vi "New.vi"(8 "error in (no error)":errorcluster, 11 "reference in":refnum<class "TestSuite_InterfaceDelegation.lvclass">) -> (0 "error out":errorcluster, 3 "reference out":refnum<class "TestSuite_InterfaceDelegation.lvclass">)   [LabVIEW 2013, in "TestSuite_InterfaceDelegation.lvclass"]
uses:
  TestSuite_InterfaceDelegation.lvclass
  Test Cases/StringList_Delegations/StringList_Delegations.lvclass
  Test Cases/ObjectList_Delegations/ObjectList_Delegations.lvclass
  <vilib>/addons/_JKI Toolkits/VI Tester/TestCase.llb/TestCase.lvclass
  TestSuite_InterfaceDelegation.lvclass/TestSuite_InterfaceDelegation.ctl
  <vilib>/addons/_JKI Toolkits/VI Tester/TestSuite.llb/TestSuite.lvclass
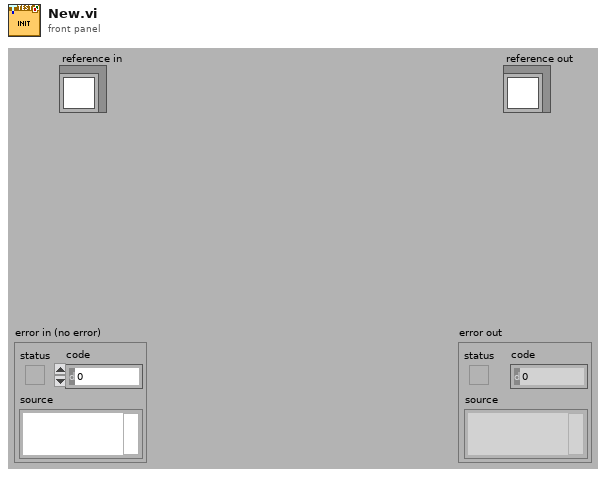
[diagram p1: front panel]
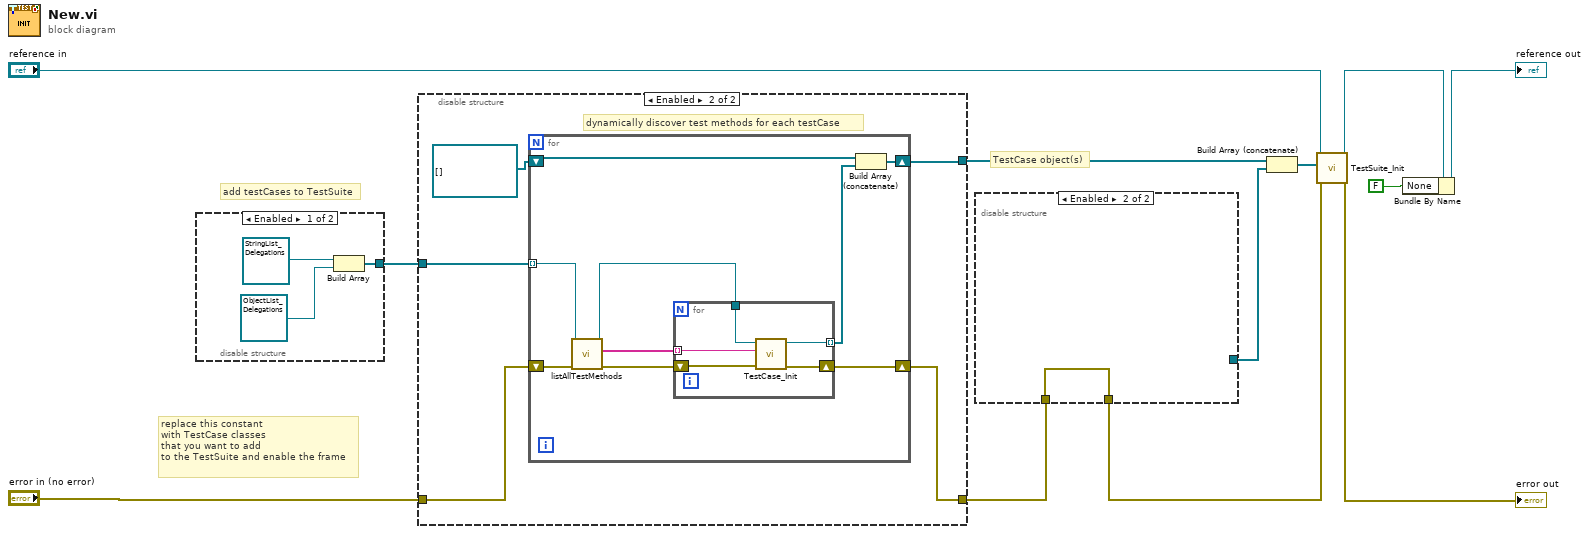
[diagram p0: block diagram]
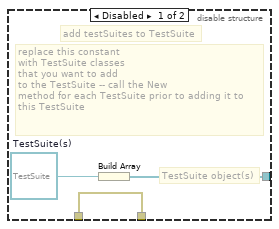
[diagram p3: hidden frame]
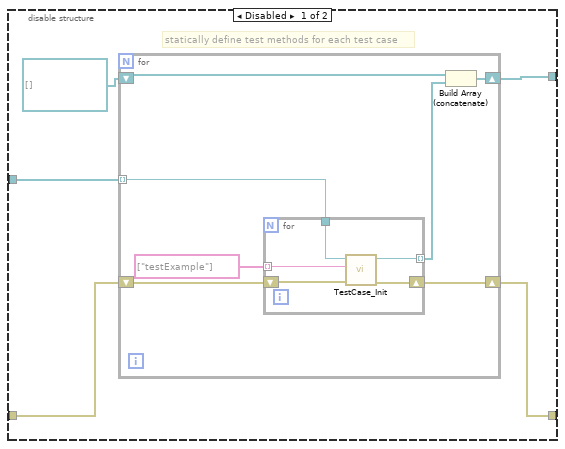
[diagram p4: hidden frame]
diagram:
  # "replace this constant\nwith TestCase classes\nthat you want to add\nto the TestSuite and enable the frame"
  # "TestCase object(s)"
  # "add testCases to TestSuite"
  n1 = disable-structure shown="Enabled" {
    disable-tunnel: [w15 _] -> w6
    frame Enabled {
      n2 = Build Array(refnum<class "StringList_Delegations.lvclass"> refnum ("StringList_Delegations.lvclass"), refnum<class "ObjectList_Delegations.lvclass"> refnum ("ObjectList_Delegations.lvclass")) -> (w15:refnum<class "TestCase.lvclass">[])
    }
    frame Disabled {
    }
  }
  n3 = disable-structure shown="Enabled" {
    disable-tunnel: w6 -> [w20 w37]
    disable-tunnel: "error in (no error)" -> [w18 w35]
    disable-tunnel: [w17 w34] -> w5
    disable-tunnel: [w16 w33] -> w1
    frame Disabled {
      # "statically define test methods for each test case"
      n4 = for {
        shift-right: [w25] -> w16
        shift-left: w18 -> [w26]
        tunnel: w20 -> [w24] mode=indexing
        shift-right: [w21] -> w17
        shift-left: refnum<class "TestCase.lvclass">[] [] -> [w22]
        n5 = for {
          tunnel: w24 -> [w28]
          tunnel: string[] ["testExample"] ("tests") -> [w32] mode=indexing
          shift-right: [w30] -> w25
          shift-left: w26 -> [w31]
          tunnel: [w29] -> w23 mode=indexing
          n6 = call <vilib>:"TestCase_Init.vi"("error in (no error)"=w31, "methodName (\"runTest\")"=w32, "TestCase in"=w28) -> ("error out"=w30:errorcluster, "TestCase out"=w29:refnum<class "TestCase.lvclass">)  [unwired: 7 in]
        }
        n7 = Build Array (concatenate)(w22, w23) -> (w21:refnum<class "TestCase.lvclass">[])
      }
    }
    frame Enabled {
      # "dynamically discover test methods for each testCase"
      n8 = for {
        shift-right: [w46] -> w33
        shift-left: w35 -> [w42]
        tunnel: w37 -> [w39] mode=indexing
        shift-right: [w43] -> w34
        shift-left: refnum<class "TestCase.lvclass">[] [] -> [w44]
        n9 = call-dynamic "listAllTestMethods.vi"("error in (no error)"=w42, "TestCase in"=w39) -> ("error out"=w41:errorcluster, "test methods"=w40:string[], "TestCase out"=w38:refnum<class "TestCase.lvclass">)  [unwired: 7 in]
        n10 = for {
          tunnel: w38 -> [w47]
          tunnel: w40 -> [w51] mode=indexing
          shift-right: [w49] -> w46
          shift-left: w41 -> [w50]
          tunnel: [w48] -> w45 mode=indexing
          n11 = call <vilib>:"TestCase_Init.vi"("error in (no error)"=w50, "methodName (\"runTest\")"=w51, "TestCase in"=w47) -> ("error out"=w49:errorcluster, "TestCase out"=w48:refnum<class "TestCase.lvclass">)  [unwired: 7 in]
        }
        n12 = Build Array (concatenate)(w44, w45) -> (w43:refnum<class "TestCase.lvclass">[])
      }
    }
  }
  n13 = disable-structure shown="Enabled" {
    disable-tunnel: [w52 _] -> w3
    disable-tunnel: [w54 w55] -> w2
    disable-tunnel: w1 -> [w54 w55]
    frame Disabled {
      w53 = refnum<class "TestSuite.lvclass"> refnum  # TestSuite(s)
      # "replace this constant\nwith TestSuite classes\nthat you want to add\nto the TestSuite -- call the New\nmethod for each TestSuite prior to adding it to\nthis TestSuite"
      # "add testSuites to TestSuite"
      # "TestSuite object(s)"
      n14 = Build Array(w53) -> (w52:refnum<class "TestSuite.lvclass">[])
    }
    frame Enabled {
    }
  }
  n15 = Build Array (concatenate)(w5, w3) -> (w4:refnum<class>[])
  n16 = call <vilib>:"TestSuite_Init.vi"("error in (no error)"=w2, "tests (none)"=w4, "TestSuite in"="reference in") -> ("error out"=→"error out":errorcluster, "TestSuite out"=w7:refnum<class "TestSuite_InterfaceDelegation.lvclass">)  [unwired: 7 in]
  n17 = Bundle By Name(cluster=w7, "None"=FALSE) -> (→"reference out":refnum<class "TestSuite_InterfaceDelegation.lvclass">)
